vi "Edit Configuration File.vi"(11 "error in (no error)":errorcluster) -> (15 "error out":errorcluster)   [LabVIEW 2021]
uses:
  <vilib>/Utility/sysdir.llb/System Directory Type.ctl
  <vilib>/Utility/config.llb/Write Key (String).vi
  <vilib>/Utility/config.llb/NI_LVConfig.lvlib
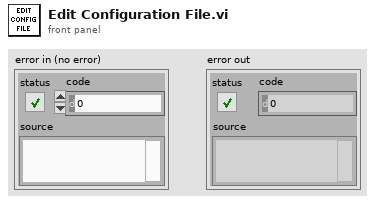
[diagram p1: front panel]
types:
  T1 = typedef "System Directory Type.ctl" = i32
  T2 = typedef "NI_LVConfig.lvlib/Config Data RefNum.ctl" = refnum<k1>
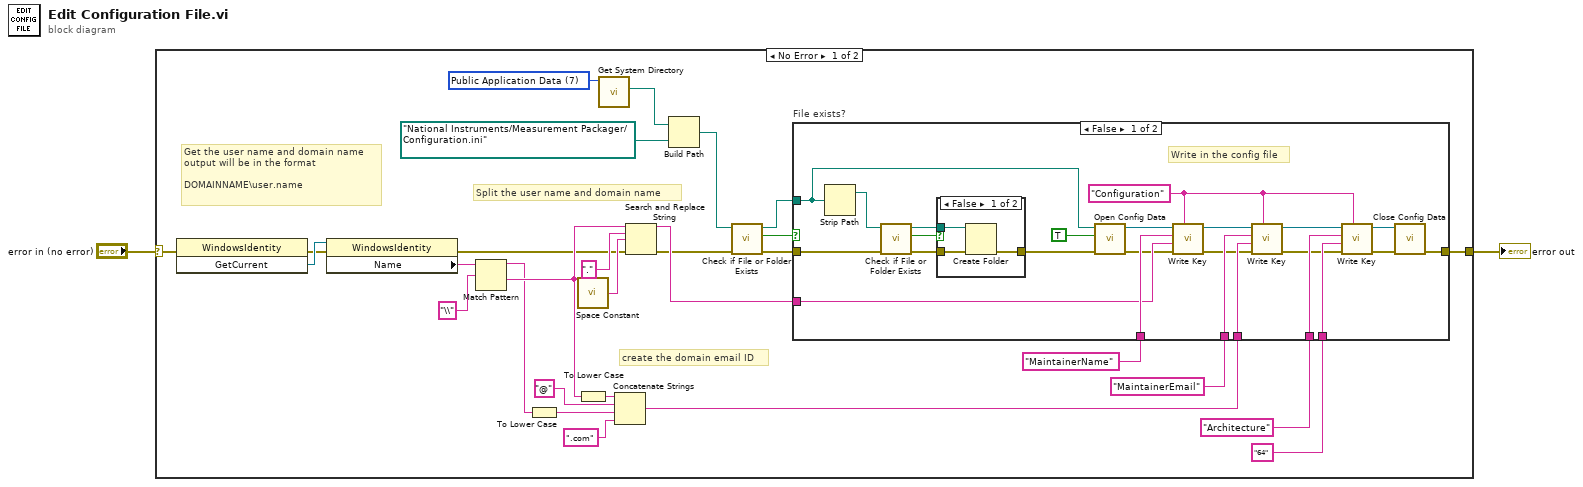
[diagram p0: block diagram]
diagram:
  n1 = case shown="No Error" "error in (no error)" {
    selector: "error in (no error)" -> [w9 w61]
    tunnel: [w4 w61] -> w1
    frame No Error {
      w3 = T1 7 items=["User Home"=0, "User Desktop"=1, "User Documents"=2, "User Application Data"=3, "User Preferences"=4, "User Temporary"=5, "Public Documents"=6, "Public Application Data"=7, "Public Preferences"=8, "Public Cache"=13, "System Core Libraries"=9, "System Installed Libraries"=10, "Application Files"=11, "Boot Volume Root"=12] ("system directory type")
      # "create the domain email ID"
      # "Split the user name and domain name"
      # "Get the user name and domain name\noutput will be in the format\n\nDOMAINNAME\\user.name"
      n2 = invoke class="WindowsIdentity" method="GetCurrent"(error in=w9) -> (error out=w8:errorcluster, "GetCurrent"=w31:refnum<k24>)  [unwired: 2 in, 1 out]
      n3 = property class="WindowsIdentity"(reference=w31, error in=w8) -> (error out=w7:errorcluster, "Name"=w29:string)  [unwired: 1 out]
      n4 = Match Pattern(string=w29, regular expression="\\") -> (before substring=w23:string, after substring=w25:string)  [unwired: 1 in, 2 out]
      n5 = To Lower Case(string=w23) -> (all lower case string=w22:string)
      n6 = call <vilib>:"Space Constant.vi"() -> ("String"=w27:string)
      n7 = To Lower Case(string=w25) -> (all lower case string=w18:string)
      n8 = call <vilib>:"Get System Directory.vi"("system directory type"=w3) -> ("system directory"=w12:path)  [unwired: 10 in]
      n9 = Concatenate Strings(w18, "@" ("string"), w22, ".com" ("string")) -> (w21:string)
      n10 = Search and Replace String(input string=w25, search string=".", replace string=w27, error in=w7) -> (result string=w20:string, error out=w6:errorcluster)  [unwired: 4 in, 2 out]
      n11 = Build Path(base path=w12, name or relative path=path "National Instruments/Measurement Packager/Configuration.ini") -> (appended path=w15:path)
      n12 = call <vilib>:"Check if File or Folder Exists.vi"("error in (no error)"=w6, "path"=w15) -> ("error out"=w5:errorcluster, "file or folder exists?"=w19:bool, "dup path"=w14:path)  [unwired: 7 in]
      n13 = case "File exists?" shown="False" w19 {
        tunnel: "MaintainerName" ("section") -> [w53 _]
        tunnel: "MaintainerEmail" ("section") -> [w52 _]
        tunnel: w21 -> [w51 _]
        tunnel: w20 -> [w50 _]
        tunnel: "Architecture" ("section") -> [w46 _]
        tunnel: "64" ("section") -> [w45 _]
        tunnel: w14 -> [w33 _]
        tunnel: w5 -> [w43 w60]
        tunnel: [w34 w60] -> w4
        frame False {
          w32 = "Configuration" ("section")
          # "Write in the config file"
          n14 = Strip Path(path=w33) -> (stripped path=w44:path)  [unwired: 1 out]
          n15 = call <vilib>:"Check if File or Folder Exists.vi"("error in (no error)"=w43, "path"=w44) -> ("error out"=w42:errorcluster, "file or folder exists?"=w40:bool, "dup path"=w41:path)  [unwired: 7 in]
          n16 = case shown="False" w40 {
            tunnel: w42 -> [w58 w59]
            tunnel: w41 -> [w57 _]
            tunnel: [w56 w59] -> w39
            frame False {
              n17 = Create Folder(path (use dialog)=w57, error in=w58) -> (error out=w56:errorcluster)  [unwired: 1 in, 2 out]
            }
            frame True {
            }
          }
          n18 = call <vilib>:"Open Config Data.vi"("error in (no error)"=w39, "create file if necessary (T)"=TRUE, "configuration file path"=w33) -> ("error out"=w38:errorcluster, "refnum"=w55:T2)  [unwired: 6 in, 1 out]
          n19 = call-poly <vilib>:"Write Key.vi"("section"=w32, "error in (no error)"=w38, "value"=w50, "key"=w53, "refnum"=w55) -> ("error out"=w37:errorcluster, "refnum out"=w54:T2)  [unwired: 4 in, 1 out]
          n20 = call-poly <vilib>:"Write Key.vi"("section"=w32, "error in (no error)"=w37, "value"=w51, "key"=w52, "refnum"=w54) -> ("error out"=w36:errorcluster, "refnum out"=w48:T2)  [unwired: 4 in, 1 out]
          n21 = call-poly <vilib>:"Write Key.vi"("section"=w32, "error in (no error)"=w36, "value"=w45, "key"=w46, "refnum"=w48) -> ("error out"=w35:errorcluster, "refnum out"=w47:T2)  [unwired: 4 in, 1 out]
          n22 = call <vilib>:"Close Config Data.vi"("error in (no error)"=w35, "refnum"=w47) -> ("error out"=w34:errorcluster)  [unwired: 8 in, 1 out]
        }
        frame True {
        }
      }
    }
    frame Error {
    }
  }
  "error out" <- w1
